vi "GenerateEventUpdateList.vi"(9 "ProjectItem":refnum<class "ProjectItem.lvclass">, 11 "UpdateList":T1) -> ()   [LabVIEW 2019, in "SolutionBuilder.lvlib" / "ProjectItem.lvclass"]
uses:
  ProjectItem.lvclass
  Events/EventUpdateList.ctl
  ProjectItem.lvclass/ProjectItem.ctl
  SolutionBuilder.lvlib
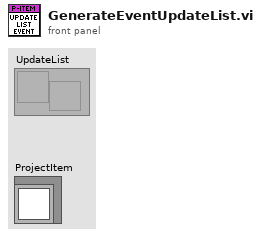
[diagram p1: front panel]
types:
  T1 = typedef "SolutionBuilder.lvlib/EventUpdateList.ctl" = refnum<user-event>
  T2 = cluster{"Build spec name":string, "Target":string, "Owning lib name":string, "name":string}
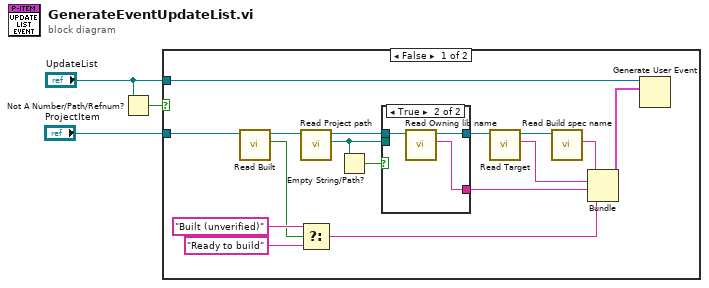
[diagram p0: block diagram]
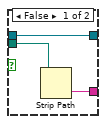
[diagram p2: hidden frame]
diagram:
  n1 = Not A Number/Path/Refnum?(number/path/refnum="UpdateList") -> (NaN/Path/Refnum?=w1:bool)
  n2 = case shown="False" w1 {
    tunnel: "ProjectItem" -> [w19 _]
    tunnel: "UpdateList" -> [w13 _]
    frame False {
      n3 = call-dynamic "Read Built.vi"("ProjectItem in"=w19) -> ("Built"=w10:bool, "ProjectItem out"=w4:refnum<class "ProjectItem.lvclass">)  [unwired: 9 in]
      n4 = call-dynamic "Read Project path.vi"("ProjectItem in"=w4) -> ("Project path"=w8:path, "ProjectItem out"=w9:refnum<class "ProjectItem.lvclass">)  [unwired: 9 in]
      n5 = Select(t="Built (unverified)" ("name"), s=w10, f="Ready to build" ("name")) -> (s? t:f=w15:string)
      n6 = Empty String/Path?(string/path=w8) -> (empty?=w7:bool)
      n7 = case shown="True" w7 {
        tunnel: w9 -> [w21 w25]
        tunnel: [w22 w23] -> w6
        tunnel: [w21 w24] -> w5
        tunnel: w8 -> [w20 _]
        frame False {
          n8 = Strip Path(path=w20) -> (name=w22:string)  [unwired: 1 out]
        }
        frame True {
          n9 = call-dynamic "Read Owning lib name.vi"("ProjectItem in"=w25) -> ("Owning lib name"=w23:string, "ProjectItem out"=w24:refnum<class "ProjectItem.lvclass">)  [unwired: 9 in]
        }
      }
      n10 = call "Read Target.vi"("ProjectItem in"=w5) -> ("Target"=w11:string, "ProjectItem out"=w12:refnum<class "ProjectItem.lvclass">)  [unwired: 9 in]
      n11 = call-dynamic "Read Build spec name.vi"("ProjectItem in"=w12) -> ("Build spec name"=w18:string)  [unwired: 9 in, 1 out]
      n12 = Bundle("Build spec name"=w18, "Target"=w11, "Owning lib name"=w6, "name"=w15) -> (w14:T2)  [unwired: 1 in]
      n13 = Generate User Event(user event=w13, event data cluster=w14) -> ()  [unwired: 2 in, 2 out]
    }
    frame True {
    }
  }
